vi "GUI_BELLA_Plasma1_HP_Controller.vi"() -> ()   [LabVIEW 2011]
uses:
  GUI_Template/GUI_master/tcp_new_data_event.ctl
  GUI_Template/GUI_master/tcp new data cluster.ctl
panel:
  in  "PressureReading2":dbl=0.001 caption="Pressure Reading Plasma1 LP" min=-10.0 max=20.0 format="%_4p"
  in  "PressureReading 1":dbl=0.001 caption="Pressure Reading Plasma1 HP" min=-10.0 max=20.0 format="%_4p"
  in  "PressureSetPoint 2":dbl=0.001 caption="Pressure Set Point Plasma1 LP" min=0.0 max=20.0 format="%_4f"
  in  "PressureSetPoint1":dbl=0.001 caption="Pressure Set Point Plasma1 HP" min=0.0 max=20.0 format="%_4f"
  in  "GaugeEnable::1":enum16{"off", "on"}(ring) caption="GaugeEnable"
  in  "GaugeReading.device 3::1":dbl=0.001 caption="Gauge Reading Plasma1" min=-10.0 max=20.0 format="%_4p"
  in  "PressureSetPoint.device 2::1":dbl=0.001 caption="Pressure Set Point Plasma1 LP" min=0.0 max=20.0 format="%_4f"
  in  "PressureReading.device 2::1":dbl=0.001 caption="Pressure Reading Plasma1 LP" min=-10.0 max=20.0 format="%_4p"
  in  "stop":bool
  in  "PressureSetPoint.device 1::1":dbl=0.001 caption="Pressure Set Point Plasma1 HP" min=0.0 max=300.0 format="%_4f"
  in  "PressureReading.device 1::1":dbl=0.001 caption="Pressure Reading Plasma1 HP" min=-10.0 max=20.0 format="%_4p"
  in  "GUIdevice 1":string="BELLA_Plasma1_Controllers"
  out "tcp data event":T1
  out "error IO 2":errorcluster
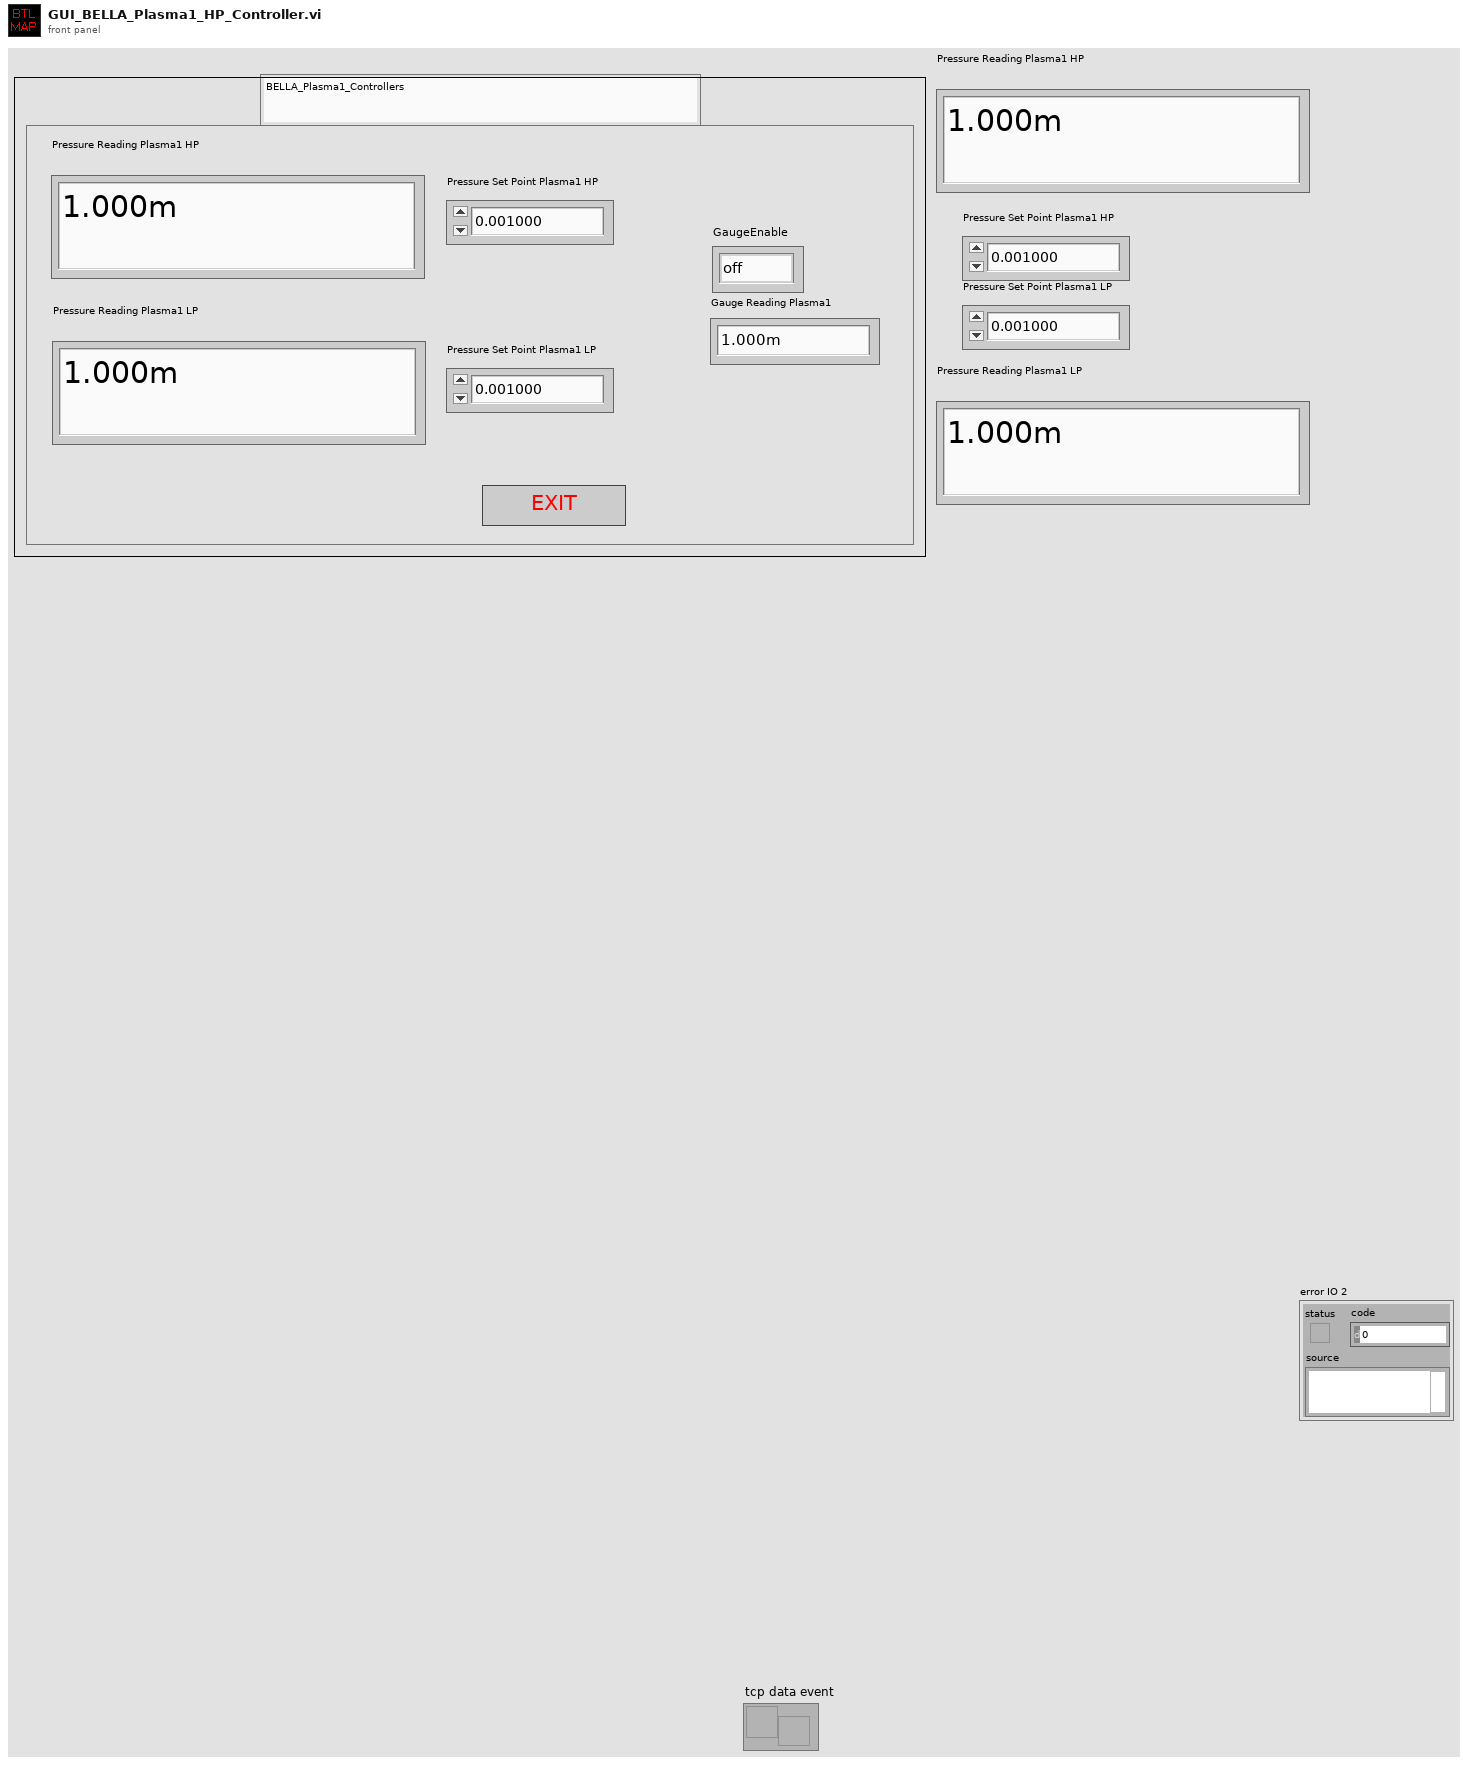
[diagram p1: front panel]
types:
  T1 = typedef "tcp_new_data_event.ctl" = refnum<user-event>
  T2 = typedef "tcp new data cluster.ctl" = cluster{"EventEnum":enum16{"new data", "connection status update"}, "Device name":string}
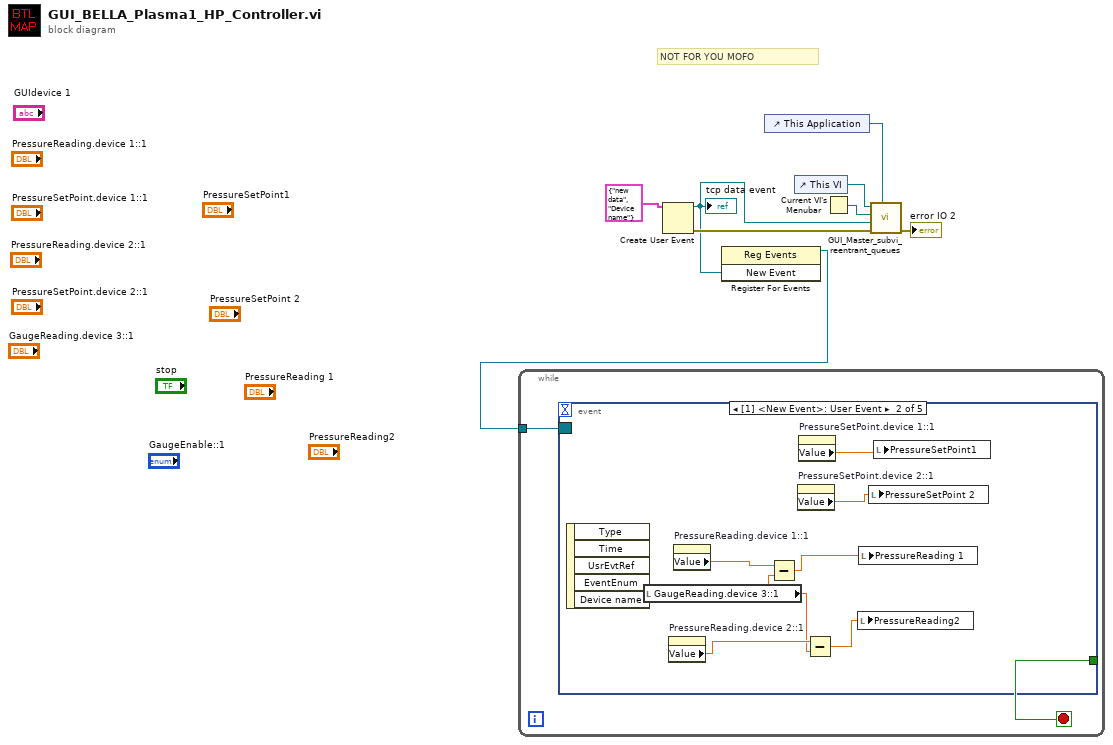
[diagram p0: block diagram]
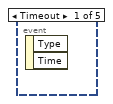
[diagram p2: hidden frame]
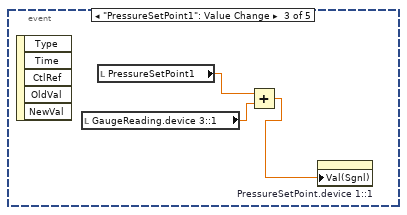
[diagram p3: hidden frame]
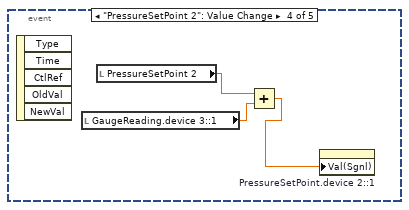
[diagram p4: hidden frame]
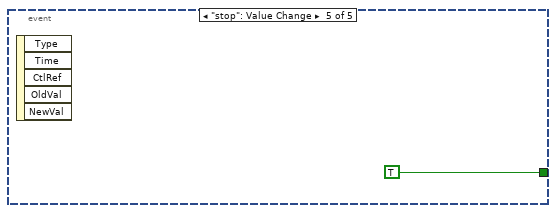
[diagram p5: hidden frame]
diagram:
  # "NOT FOR YOU MOFO"
  n1 = Create User Event(user event datatype=T2 {"EventEnum"=enum."new data", "Device name"="Device name"} ("New Event")) -> (user event=w3:refnum<user-event>, error out=w4:errorcluster)  [unwired: 1 in]
  "tcp data event" <- w3
  n2 = register-events(w3) -> (reference out=w1:refnum<event-registration>)  [unwired: 2 in, 1 out]
  n3 = while {
    tunnel: w1 -> [w10]
    stop <- w9 stop-if-true
    n4 = event shown="[1] <New Event>: User Event" {
      selector: w10 -> [_ _ _ _ _]
      dyn-events: _ -> [_ _ _ _ _]
      timeout: _ -> [_ _ _ _ _]
      tunnel: [_ _ _ _ TRUE] -> w9
      event Timeout {
        n5 = event-data() -> ()  [unwired: 1 in, 2 out]
      }
      event User Event {
        n6 = event-data() -> ()  [unwired: 1 in, 5 out]
        n7 = local read "GaugeReading.device 3::1"() -> (w13:dbl)
        n8 = property on="PressureReading.device 2::1" class="DigNum (strict)"() -> ("Value"=w15:dbl)  [unwired: 2 in, 2 out]
        n9 = property on="PressureReading.device 1::1" class="DigNum (strict)"() -> ("Value"=w17:dbl)  [unwired: 2 in, 2 out]
        n10 = Subtract(x=w17, y=w13) -> (x-y=w16:dbl)
        n11 = property on="PressureSetPoint.device 2::1" class="DigNum (strict)"() -> ("Value"=w11:dbl)  [unwired: 2 in, 2 out]
        n12 = property on="PressureSetPoint.device 1::1" class="DigNum (strict)"() -> ("Value"=w12:dbl)  [unwired: 2 in, 2 out]
        n13 = Subtract(x=w15, y=w13) -> (x-y=w14:dbl)
        n14 = local write "PressureReading2"(w14) -> ()
        n15 = local write "PressureReading 1"(w16) -> ()
        n16 = local write "PressureSetPoint 2"(w11) -> ()
        n17 = local write "PressureSetPoint1"(w12) -> ()
      }
      event "PressureSetPoint1": Value Change {
        n18 = event-data() -> ()  [unwired: 1 in, 5 out]
        n19 = local read "GaugeReading.device 3::1"() -> (w19:dbl)
        n20 = local read "PressureSetPoint1"() -> (w20:dbl)
        n21 = Add(x=w20, y=w19) -> (x+y=w18:dbl)
        n22 = property on="PressureSetPoint.device 1::1" class="DigNum (strict)"("Val(Sgnl)"=w18) -> ()  [unwired: 2 in, 2 out]
      }
      event "PressureSetPoint 2": Value Change {
        n23 = event-data() -> ()  [unwired: 1 in, 5 out]
        n24 = local read "GaugeReading.device 3::1"() -> (w22:dbl)
        n25 = local read "PressureSetPoint 2"() -> (w23:dbl)
        n26 = Add(x=w23, y=w22) -> (x+y=w21:dbl)
        n27 = property on="PressureSetPoint.device 2::1" class="DigNum (strict)"("Val(Sgnl)"=w21) -> ()  [unwired: 2 in, 2 out]
      }
      event "stop": Value Change {
        n28 = event-data() -> ()  [unwired: 1 in, 5 out]
      }
    }
  }
  n29 = control-ref of="This Application"() -> (w2:refnum<vi>)
  n30 = control-ref of="This VI"() -> (w7:refnum<vi>)
  n31 = Current VI's Menubar() -> (w6:refnum<k9>)
  n32 = call "GUI_Master_subvi_reentrant_queues.vi"("This Application"=w2, "error in (no error)"=w4, "tcp data event"=w3, "Caller menu reference"=w6, "Caller VI ref"=w7) -> ("error out"=→"error IO 2":errorcluster)  [unwired: 6 in]
